vi "CheckLiveUpdates.vi"(8 "error in (no error)":errorcluster, 9 "GraphName":string, 11 "Gserver in":refnum<class "Gserver.lvclass">) -> (0 "error out":errorcluster, 1 "index":i32, 3 "Gserver out":refnum<class "Gserver.lvclass">)   [LabVIEW 2020, in "Sgraph_lib_V1.lvlib" / "Gserver.lvclass"]
doc: "Andre Koelewijn, 17 jan 2021\n\nCheck if Live update action is present for this Gviewer"
uses:
  Gserver.lvclass
  Gserver.lvclass/Gserver.ctl
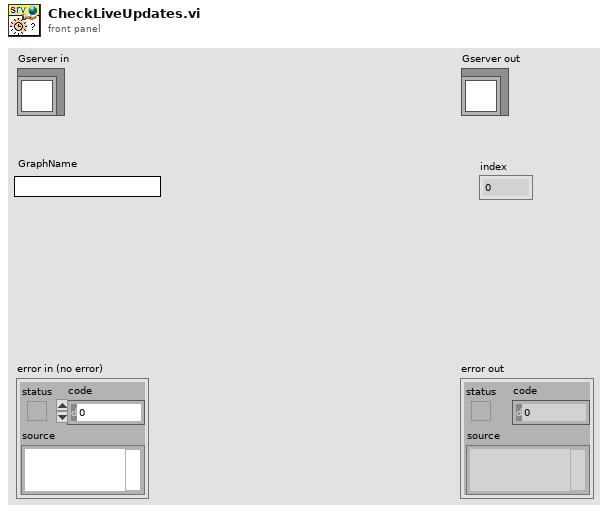
[diagram p1: front panel]
types:
  T1 = typedef "Sgraph_lib_V1.lvlib/Gserver.lvclass/Typedef_PeriodicUpdate.ctl" = cluster{"Sending Gviewer":string, "PreviousUpdate":timestamp, "UpdateRate":dbl, "DataRequest":T2}
  T2 = typedef "Sgraph_lib_V1.lvlib/Gviewer.lvclass/Typedef_datarequest.ctl" = cluster{"Tags":string[], "Live":T3, "Time-Start":timestamp, "Time-End":timestamp, "TimeSpan":dbl, "DisplayResolution":i32}
  T3 = typedef "Sgraph_lib_V1.lvlib/Gviewer.lvclass/Typedef_Live.ctl" = enum16{"Live View", "Freeze"}
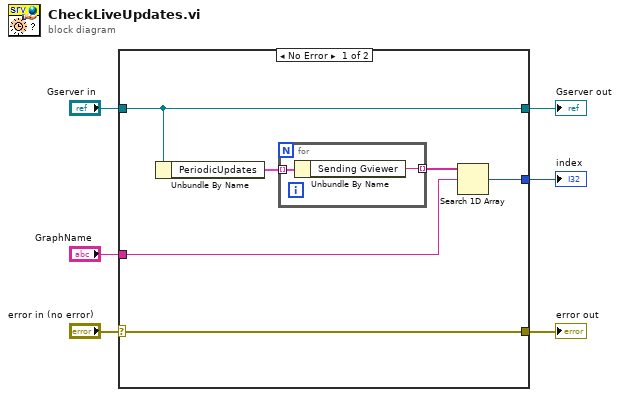
[diagram p0: block diagram]
diagram:
  n1 = case shown="No Error" "error in (no error)" {
    selector: "error in (no error)" -> [w12 w16]
    tunnel: [w12 w16] -> w5
    tunnel: [w11 w15] -> w3
    tunnel: "Gserver in" -> [w11 w15]
    tunnel: "GraphName" -> [w8 _]
    tunnel: [w7 _] -> w1
    frame No Error {
      n2 = Unbundle By Name(w11) -> ("PeriodicUpdates"=w10:T1[])
      n3 = for {
        tunnel: w10 -> [w14] mode=indexing
        tunnel: [w13] -> w9 mode=indexing
        n4 = Unbundle By Name(w14) -> ("Sending Gviewer"=w13:string)
      }
      n5 = Search 1D Array(1D array=w9, element=w8) -> (index of element=w7:i32)  [unwired: 1 in]
    }
    frame Error {
    }
  }
  "error out" <- w5
  "Gserver out" <- w3
  "index" <- w1
